vi "Set Legend (XYGraph).vi"(6 "initialize":bool, 8 "error in (no error)":errorcluster, 9 "Plot.Plot Name":string, 10 "Active Plot":i32, 11 "XYGraph in":refnum<vi>) -> (0 "error out":errorcluster, 1 "Plot.Plot Name":string, 2 "Active Plot":i32, 3 "XYGraph out":refnum<vi>)   [LabVIEW 2019, in "Instrument.Lockin.UI.lvclass"]
uses:
  Instrument.Lockin.UI.lvclass
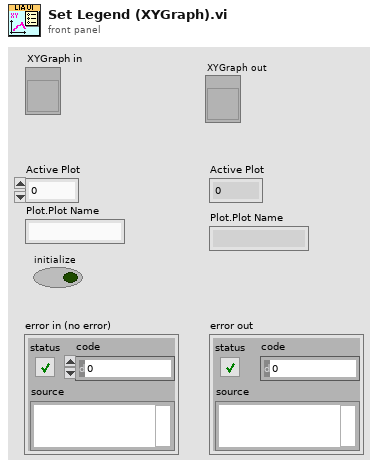
[diagram p1: front panel]
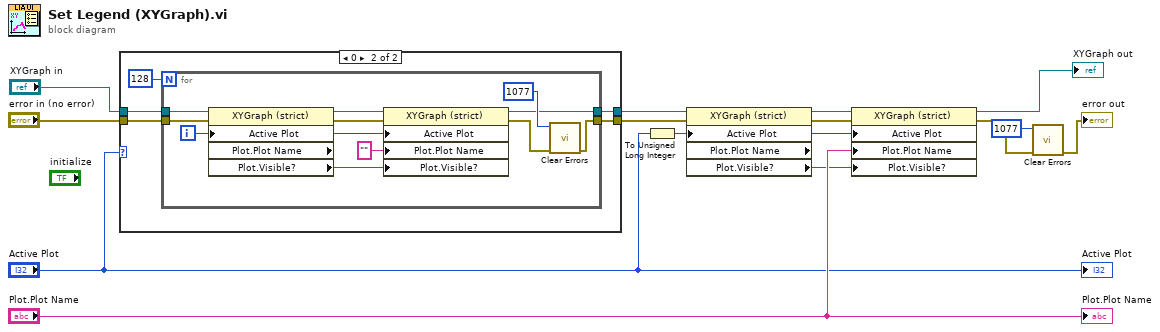
[diagram p0: block diagram]
diagram:
  n1 = case shown="0" "Active Plot" {
    tunnel: "XYGraph in" -> [w15 w18]
    tunnel: [w16 w21] -> w6
    tunnel: "error in (no error)" -> [w16 w20]
    tunnel: [w15 w17] -> w7
    frame Default {
    }
    frame 0 {
      n2 = for {
        N: 128 -> [_]
        tunnel: w18 -> [w25]
        tunnel: [w30] -> w21
        tunnel: w20 -> [w24]
        tunnel: [w28] -> w17
        i -> [w23]
        n3 = property on="Property Node" class="XYGraph (strict)" props=["Active Plot", "Plot", "Plot Name", "Plot", "Visible?"](reference=w25, error in=w24, "Active Plot"=w23) -> (reference out=w27:refnum<vi>, error out=w26:errorcluster, "Plot.Visible?"=w22:bool)  [unwired: 1 out]
        n4 = property on="Property Node" class="XYGraph (strict)"(reference=w27, error in=w26, "Active Plot"=w23, "Plot.Plot Name"="" ("format string"), "Plot.Visible?"=w22) -> (reference out=w28:refnum<vi>, error out=w31:errorcluster)
        n5 = call <vilib>:"Clear Errors.vi"("error in (no error)"=w31, "specific error code to clear (0: all)"=1077) -> ("error out"=w30:errorcluster)  [unwired: 4 in, 1 out]
      }
    }
  }
  n6 = To Unsigned Long Integer(number="Active Plot") -> (unsigned 32bit integer=w3:u32)
  n7 = property on="Property Node" class="XYGraph (strict)" props=["Active Plot", "Plot", "Plot Name", "Plot", "Visible?"](reference=w7, error in=w6, "Active Plot"=w3) -> (reference out=w5:refnum<vi>, error out=w4:errorcluster, "Plot.Visible?"=w2:bool)  [unwired: 1 out]
  n8 = property on="Property Node" class="XYGraph (strict)"(reference=w5, error in=w4, "Active Plot"=w3, "Plot.Plot Name"="Plot.Plot Name", "Plot.Visible?"=w2) -> (reference out=→"XYGraph out":refnum<vi>, error out=w13:errorcluster)
  n9 = call <vilib>:"Clear Errors.vi"("error in (no error)"=w13, "specific error code to clear (0: all)"=1077) -> ("error out"=→"error out":errorcluster)  [unwired: 4 in, 1 out]
  "Active Plot" <- "Active Plot"
  "Plot.Plot Name" <- "Plot.Plot Name"
